vi "lab3.vi"() -> ()   [LabVIEW 2023]
uses:
  200f3d78-f65f-466c-b6b3-4ed96b6c02ea.vi
  <vilib>/Array/Sort 2D Array - Pop Stack.vi
  <vilib>/Array/Sort 2D Array - Push Stack.vi
  200f3d78-f65f-466c-b6b3-4ed96b6c02ea.vi/269d4b3b-47f5-49e3-8884-44851e4dd9d5.vi
  200f3d78-f65f-466c-b6b3-4ed96b6c02ea.vi/6d99389c-673d-4efb-bf33-19b32bcf4cf8.vi
panel:
  out "Waveform Graph":dbl[](graph)
  out "Waveform Chart":dbl(graph)
  out "Number of iteration":i32
  out "sorted 2D array":dbl[][](array[numeric])
  out "Array with sorted rows":dbl[][](array[numeric])
  out "element (9,9)":dbl
  out "Last generated value":dbl
  out "generated array":dbl[][](array[numeric])
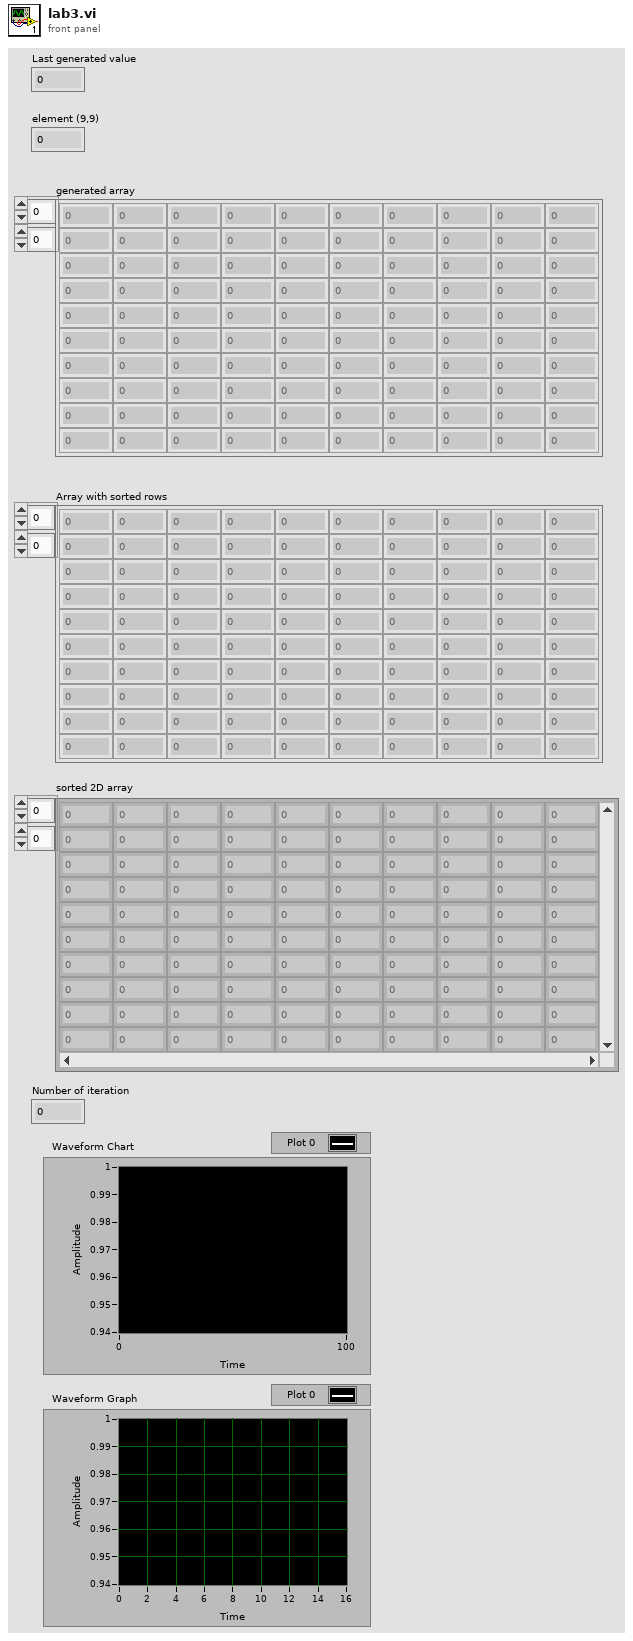
[diagram p1: front panel]
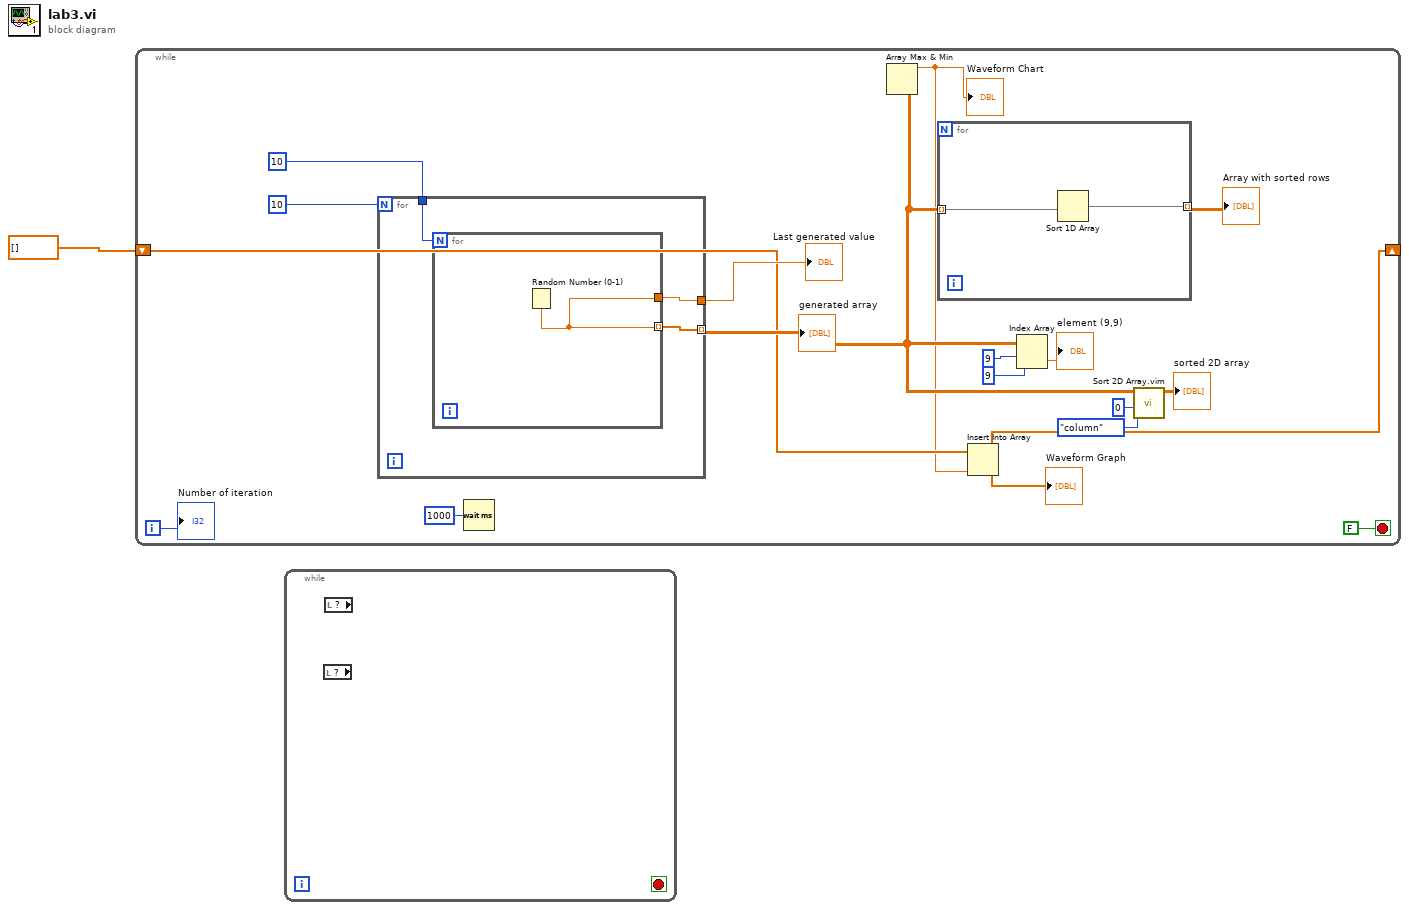
[diagram p0: block diagram]
diagram:
  n1 = while {
    shift-right: [w3] -> _
    shift-left: dbl[] [] -> [w4]
    i -> [w6]
    stop <- FALSE stop-if-true
    n2 = for {
      N: 10 -> [_]
      tunnel: 10 -> [w23]
      tunnel: [w22] -> w16
      tunnel: [w21] -> w5 mode=indexing
      n3 = for {
        N: w23 -> [_]
        tunnel: [w24] -> w22
        tunnel: [w24] -> w21 mode=indexing
        n4 = Random Number (0-1)() -> (number: 0 to 1=w24:dbl)
      }
    }
    "generated array" <- w5
    "Last generated value" <- w16
    n5 = Wait (ms)(milliseconds to wait=u32 1000) -> ()  [unwired: 1 out]
    n6 = Array Max & Min(array=w5) -> (max value=w2:dbl)  [unwired: 3 out]
    "Waveform Chart" <- w2
    n7 = for {
      tunnel: w5 -> [w20] mode=indexing
      tunnel: [w19] -> w12 mode=indexing
      n8 = Sort 1D Array(array=w20) -> (sorted array=w19:dbl[])
    }
    "Array with sorted rows" <- w12
    n9 = Insert Into Array(array=w4, new element=w2) -> (w3:dbl[])  [unwired: 1 in]
    "Waveform Graph" <- w3
    n10 = Index Array(array=w5, index (row)=9, index (col)=9) -> (element=→"element (9,9)":dbl)
    n11 = call "Sort 2D Array.vim"("index"=0, "dimension to index (column)"=enum16{"column", "row"}."column", "2D array"=w5) -> ("sorted 2D array"=→"sorted 2D array":dbl[][])  [unwired: 7 in, 1 out]
    "Number of iteration" <- w6
  }
  n12 = while {
    stop <- _ stop-if-true
    n13 = local read item#-1() -> ()  [unwired: 1 out]
    n14 = local read item#-1() -> ()  [unwired: 1 out]
  }
